vi "GetText.vi"(8 "error in":errorcluster, 11 "Temperature Controller Logic editor node in":refnum<class "Temperature Controller Logic editor node.lvclass">) -> (0 "error out":errorcluster, 1 "additional text":string, 2 "text":string, 3 "Temperature Controller Logic editor node out":refnum<class "Temperature Controller Logic editor node.lvclass">, 4 "glyph":string)   [LabVIEW 2013, in "Temperature Controller Logic editor node.lvclass"]
uses:
  Temperature Controller Logic editor node.lvclass
  <vilib>/NI/Tag Bus Data Framework/control module/editor node/control module editor.lvclass
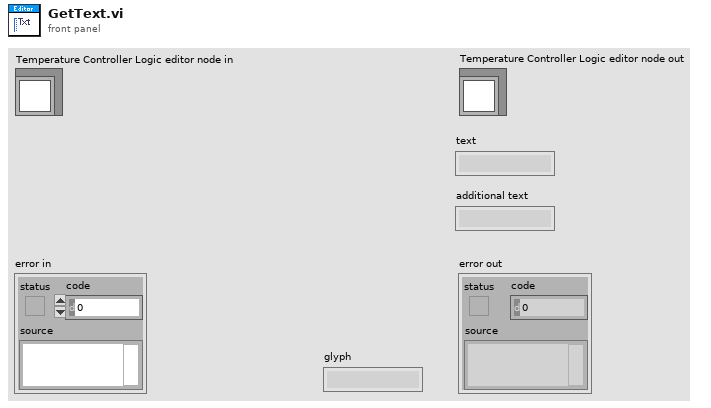
[diagram p1: front panel]
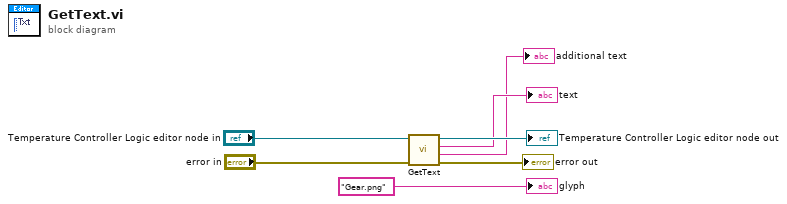
[diagram p0: block diagram]
diagram:
  n1 = call-parent "GetText.vi"("error in"="error in", "Module Editor Node in"="Temperature Controller Logic editor node in") -> ("error out"=→"error out":errorcluster, "additional text"=→"additional text":string, "text"=→"text":string, "Module Editor Node out"=→"Temperature Controller Logic editor node out":refnum<class "Temperature Controller Logic editor node.lvclass">)  [unwired: 5 in, 1 out]
  "glyph" <- "Gear.png" ("glyph")
